vi "Remove Meta.vi"(8 "error in (no error)":errorcluster, 10 "Meta Name":string, 11 "Config Element in":refnum<class "Config Element.lvclass">) -> (0 "error out":errorcluster, 2 "Removed":bool, 3 "Config Element out":refnum<class "Config Element.lvclass">)   [LabVIEW 2023, in "CDM-Config.lvlib" / "Config Element.lvclass"]
doc: "Removes a meta field from the element."
uses:
  Config Element.lvclass
  Config Element.lvclass/Config Element.ctl
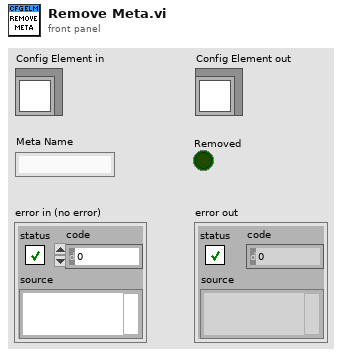
[diagram p1: front panel]
types:
  T1 = typedef "CDM-Config.lvlib/Config Element.lvclass/Element Data.ctl" = cluster{"Node Info":T2, "Owner":refnum<class>, "Changed":bool, "Name":string, "Meta Data":T3[], "Value Type":T4, "Value":variant}
  T2 = typedef "CDM-Config.lvlib/Node Info.ctl" = cluster{"Index":i32, "Parent":i32, "Children":i32[]}
  T3 = typedef "CDM-Config.lvlib/Meta Data.ctl" = cluster{"Name":string, "Value":string}
  T4 = typedef "CDM-Config.lvlib/Value Type.ctl" = enum16{"String", "Number", "Bool", "Object", "Array"}
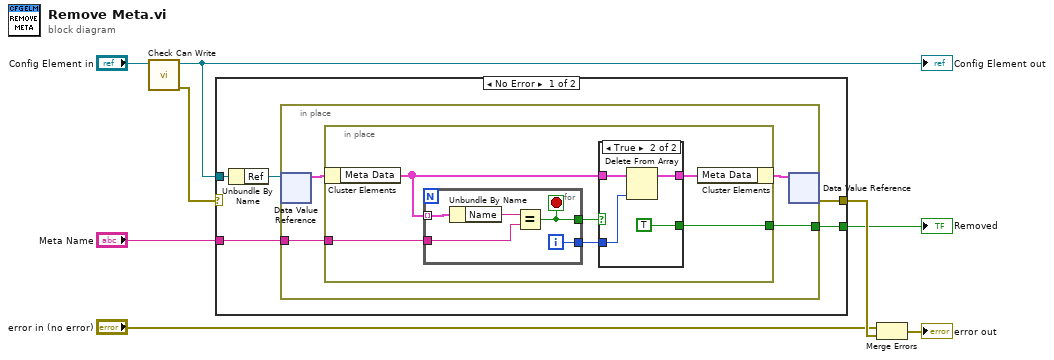
[diagram p0: block diagram]
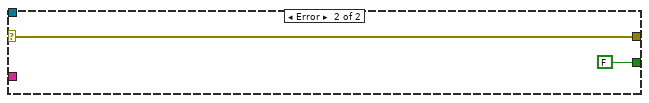
[diagram p3: hidden frame]
diagram:
  n1 = call "Check Can Write.vi"("Config Element in"="Config Element in") -> ("error out"=w1:errorcluster, "Config Element out"=w2:refnum<class "Config Element.lvclass">)  [unwired: 9 in]
  "Config Element out" <- w2
  n2 = case shown="No Error" w1 {
    selector: w1 -> [_ w35]
    tunnel: [w13 w35] -> w8
    tunnel: "Meta Name" -> [w11 _]
    tunnel: [w10 FALSE] -> w5
    tunnel: w2 -> [w9 _]
    frame No Error {
      n3 = Unbundle By Name(w9) -> ("Ref"=w12:refnum<data-value>)
      n4 = in-place {
        in-place-border: w11 -> [w15]
        in-place-border: [w14] -> w10
        n5 = in-place-dvr #1(w12) -> (w17:T1)  [unwired: 1 out]
        n6 = in-place {
          in-place-border: w15 -> [w21]
          in-place-border: [w18] -> w14
          n7 = in-place-cluster #2(w17) -> ("Meta Data"=w23:T3[])
          n8 = for {
            tunnel: w23 -> [w33] mode=indexing
            tunnel: w21 -> [w31]
            tunnel: [w30] -> w20
            tunnel: [w29] -> w19
            i -> [w29]
            stop <- w30 stop-if-true
            n9 = Unbundle By Name(w33) -> ("Name"=w32:string)
            n10 = Equal?(x=w32, y=w31) -> (x = y?=w30:bool)
          }
          n11 = case shown="True" w20 {
            tunnel: w19 -> [_ w27]
            tunnel: w23 -> [w24 w28]
            tunnel: [w24 w26] -> w22
            tunnel: [_ TRUE] -> w18
            frame False {
            }
            frame True {
              n12 = Delete From Array(array=w28, index=w27) -> (array with subset deleted=w26:T3[])  [unwired: 1 in, 1 out]
            }
          }
          n13 = in-place-cluster #2("Meta Data"=w22) -> (w16:T1)
        }
        n14 = in-place-dvr #1(w16) -> (w13:errorcluster)  [unwired: 1 out]
      }
    }
    frame Error {
    }
  }
  "Removed" <- w5
  n15 = Merge Errors("error in (no error)", w8) -> (→"error out":errorcluster)
